vi "Singleton.vi"(8 "error in (no error)":errorcluster, 10 "Close?":bool) -> (0 "error out":errorcluster)   [LabVIEW 2017, in "MGI-Console.lvlib" / "Console.lvclass"]
doc: "Stores the console reference.\n----\nCopyright: MGI 2018\nAuthor: Derek Trepanier"
uses:
  Console.lvclass
  kernel32.dll
  user32.dll
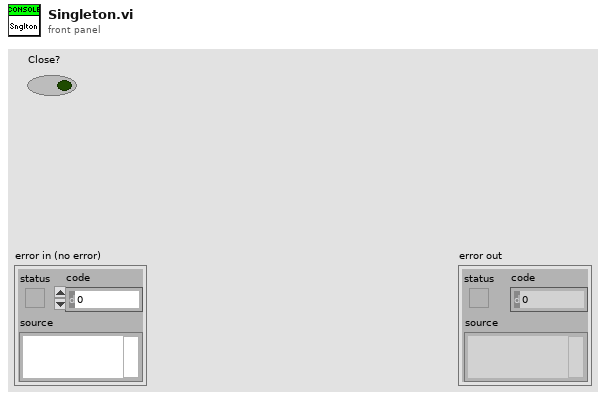
[diagram p1: front panel]
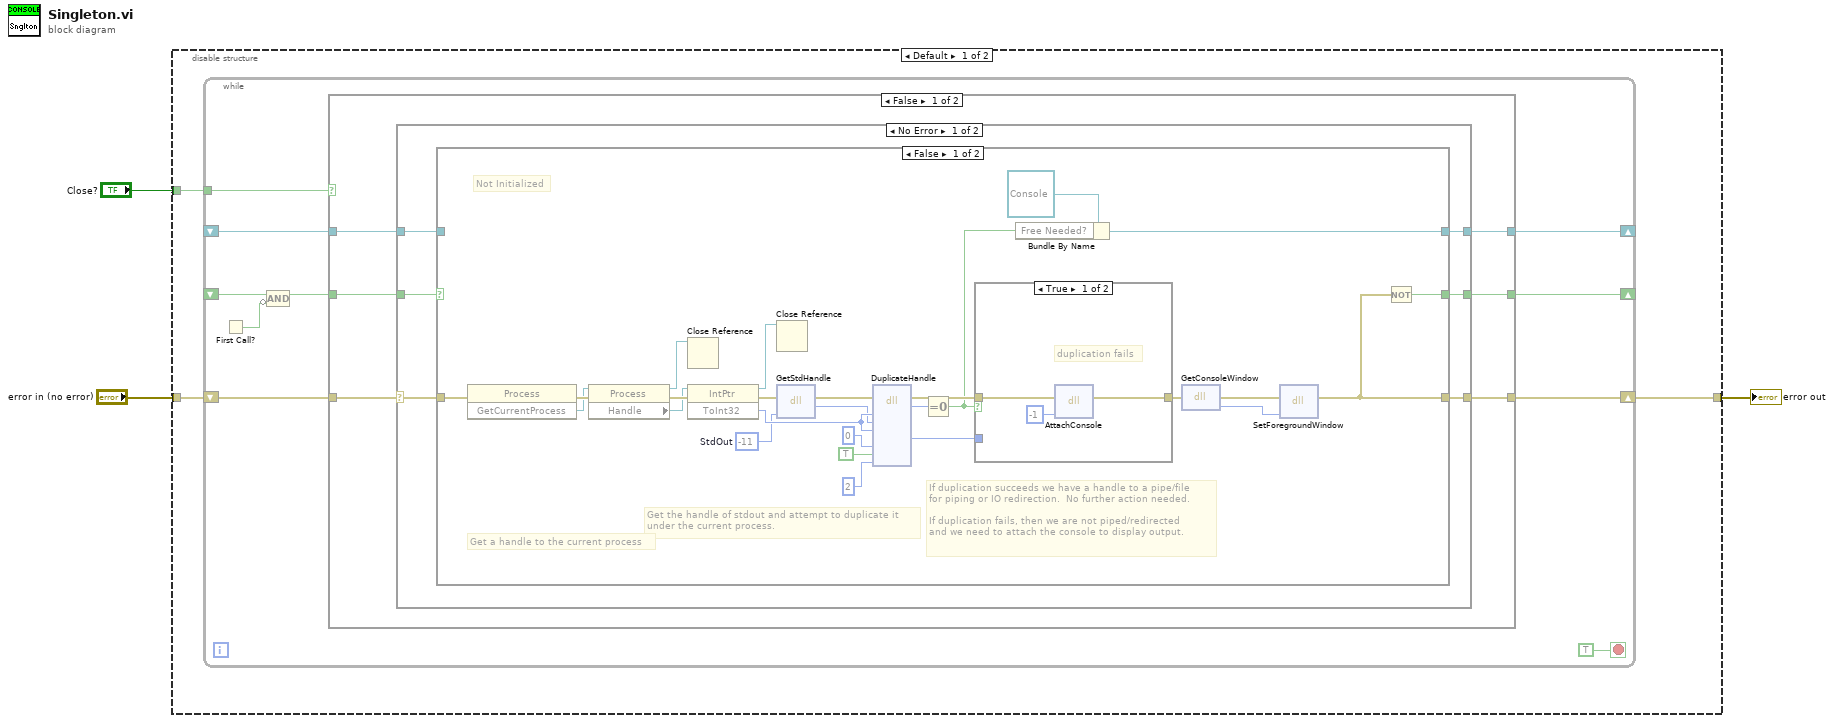
[diagram p0: block diagram]
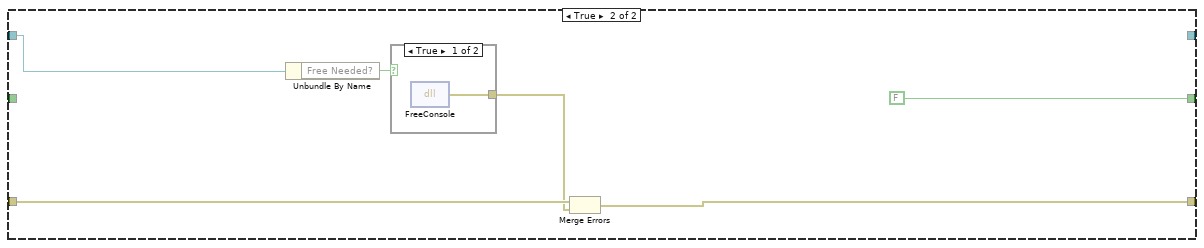
[diagram p5: hidden frame]
diagram:
  n1 = disable-structure shown="Default" {
    disable-tunnel: "error in (no error)" -> [w6 w72]
    disable-tunnel: [w5 w72] -> w2
    disable-tunnel: "Close?" -> [w4 _]
    frame condition #0 {
      n2 = while {
        shift-right: [w15] -> w5
        shift-left: w6 -> [w16]
        shift-right: [w14] -> _
        shift-left: _ -> [w12]
        tunnel: w4 -> [w11]
        shift-right: [w10] -> _
        shift-left: _ -> [w9]
        stop <- TRUE stop-if-true
        n3 = First Call?() -> (First Call?: T/F=w7:bool)
        n4 = Compound Arithmetic op=AND(w9, invert w7) -> (w8:bool)
        n5 = case shown="False" w11 {
          tunnel: w16 -> [w22 w68]
          tunnel: [w21 w67] -> w15
          tunnel: [w20 _] -> w14
          tunnel: w12 -> [w19 w69]
          tunnel: [w18 FALSE] -> w10
          tunnel: w8 -> [w17 _]
          frame False {
            n6 = case shown="No Error" w22 {
              selector: w22 -> [w28 w63]
              tunnel: [w26 w63] -> w21
              tunnel: [w27 w64] -> w20
              tunnel: w19 -> [w23 w64]
              tunnel: [w25 w62] -> w18
              tunnel: w17 -> [w24 w62]
              frame No Error {
                n7 = case shown="False" w24 {
                  selector: w24 -> [_ w61]
                  tunnel: w28 -> [w35 w60]
                  tunnel: [w34 w59] -> w27
                  tunnel: [w29 w60] -> w26
                  tunnel: [w33 w61] -> w25
                  tunnel: w23 -> [_ w59]
                  frame False {
                    w46 = -11  # StdOut
                    # "Not Initialized"
                    # "If duplication succeeds we have a handle to a pipe/file\nfor piping or IO redirection.  No further action needed.\n\nIf duplication fails, then we are not piped/redirected\nand we need to attach the console to display output."
                    # "Get the handle of stdout and attempt to duplicate it\nunder the current process."
                    # "Get a handle to the current process"
                    n8 = invoke class="Process" method="GetCurrentProcess"(error in=w35) -> (error out=w53:errorcluster, "GetCurrentProcess"=w44:refnum<k24>)  [unwired: 2 in, 1 out]
                    n9 = property class="Process"(reference=w44, error in=w53) -> (reference out=w38:refnum<k24>, error out=w52:errorcluster, "Handle"=w43:refnum<k24>)
                    n10 = Close Reference(reference=w38) -> ()  [unwired: 1 in, 1 out]
                    n11 = invoke class="IntPtr" method="ToInt32"(reference=w43, error in=w52) -> (reference out=w39:refnum<k24>, error out=w47:errorcluster, "ToInt32"=w54:i32)  [unwired: 1 in]
                    n12 = Close Reference(reference=w39) -> ()  [unwired: 1 in, 1 out]
                    n13 = dll-call lib="kernel32.dll" fn="GetStdHandle"(error in=w47, "nStdHandle"=w46) -> (error out=w42:errorcluster, "return type"=w45:i32)  [unwired: 3 in, 1 out]
                    n14 = dll-call lib="kernel32.dll" fn="DuplicateHandle"(error in=w42, "hSourceProcess"=w54, "hSourceHandle"=w45, "hTargetProcess"=w54, "dwDesirecAccess"=u16 0, "bInheritHandle"=TRUE, "dwOptions"=u16 2) -> (error out=w51:errorcluster, "return type"=w41:u8, "lpTargetHandle"=w40:i32)  [unwired: 9 in, 1 out]
                    n15 = Equal To 0?(x=w41) -> (x = 0?=w37:bool)
                    n16 = case shown="True" w37 {
                      tunnel: w51 -> [w57 w58]
                      tunnel: [w56 w58] -> w31
                      tunnel: w40 -> [_ _]
                      frame True {
                        # "duplication fails"
                        n17 = dll-call lib="kernel32.dll" fn="AttachConsole"(error in=w57, "arg1"=-1) -> (error out=w56:errorcluster)  [unwired: 4 in, 1 out]
                      }
                      frame False {
                        # "duplication succeeds"
                      }
                    }
                    n18 = Bundle By Name(cluster=refnum<class "Console.lvclass"> refnum ("Console in"), "Free Needed?"=w37) -> (w34:refnum<class "Console.lvclass">)
                    n19 = dll-call lib="kernel32.dll" fn="GetConsoleWindow"(error in=w31) -> (error out=w30:errorcluster, "return type"=w32:i64)  [unwired: 2 in, 1 out]
                    n20 = dll-call lib="user32.dll" fn="SetForegroundWindow"(error in=w30, "arg1"=w32) -> (error out=w29:errorcluster)  [unwired: 4 in, 1 out]
                    n21 = Not(x=w29) -> (.not. x?=w33:bool)
                  }
                  frame True {
                    # "Already Initialized"
                  }
                }
              }
              frame Error {
              }
            }
          }
          frame True {
            n22 = Unbundle By Name(w69) -> ("Free Needed?"=w70:bool)
            n23 = case shown="True" w70 {
              tunnel: [w71 _] -> w66
              frame True {
                n24 = dll-call lib="kernel32.dll" fn="FreeConsole"() -> (error out=w71:errorcluster)  [unwired: 3 in, 2 out]
              }
              frame False {
              }
            }
            n25 = Merge Errors(w68, w66) -> (w67:errorcluster)
          }
        }
      }
    }
    frame condition #1 (active) {
    }
  }
  "error out" <- w2
